vi "get z location.vi"(11 "tag lens trigger":bool) -> (1 "counts in last cycle":u16, 2 "fly back":bool, 3 "z location":i16)   [LabVIEW 2010]
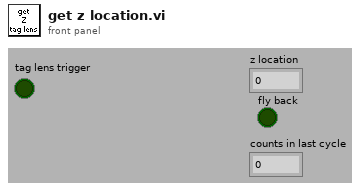
[diagram p1: front panel]
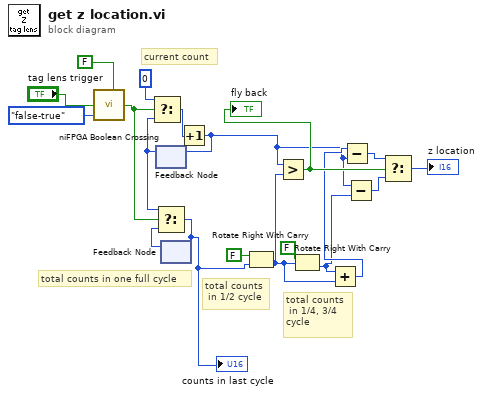
[diagram p0: block diagram]
diagram:
  # "total counts\n in 1/4, 3/4 cycle"
  # "total counts\n in 1/2 cycle"
  # "total counts in one full cycle"
  # "current count"
  n1 = call <vilib>:"niFPGA Boolean Crossing.vi"("input"="tag lens trigger", "direction"=enum8{"either", "false-true", "true-false"}."false-true", "initialize"=FALSE) -> ("crossing"=w13:bool)  [unwired: 6 in]
  n2 = feedback #1() -> (w14:u16)  [unwired: 1 in]
  n3 = Select(t=u16 0, s=w13, f=w14) -> (s? t:f=w15:u16)
  n4 = feedback #2() -> (w12:u16)  [unwired: 1 in]
  n5 = Select(t=w14, s=w13, f=w12) -> (s? t:f=w10:u16)
  "counts in last cycle" <- w10
  n6 = feedback-in #2(w10) -> ()
  n7 = Increment(x=w15) -> (x+1=w3:u16)
  n8 = feedback-in #1(w3) -> ()
  n9 = Rotate Right With Carry(2:w10, 3:FALSE ("carry")) -> (0:w8:u16)  [unwired: 1 out]
  n10 = Greater?(x=w3, y=w8) -> (0:w7:bool)
  "fly back" <- w7
  n11 = Rotate Right With Carry(2:w8, 3:FALSE ("carry")) -> (0:w4:u16)  [unwired: 1 out]
  n12 = Add(x=w4, y=w8) -> (x+y=w5:u16)
  n13 = Subtract(x=w5, y=w3) -> (x-y=w6:i16)
  n14 = Subtract(x=w3, y=w4) -> (x-y=w2:i16)
  n15 = Select(t=w6, s=w7, f=w2) -> (s? t:f=→"z location":i16)
